vi "Cap_vs_RF-power.vi"() -> ()   [LabVIEW 2020]
uses:
  <vilib>/Utility/file.llb/Write Delimited Spreadsheet (string).vi
  <instrlib>/Agilent 428X Series/Agilent 428X Series.lvlib
  <instrlib>/Agilent PSG MXG Series/Agilent PSG MXG Series.lvlib
panel:
  in  "Register arrays":string[](array[string])
  in  "file path (dialog if empty)":path
  out "error out":errorcluster
  out "Array":string[][](array[string])
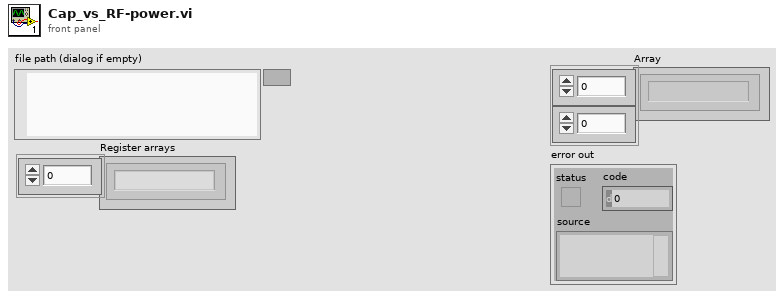
[diagram p1: front panel]
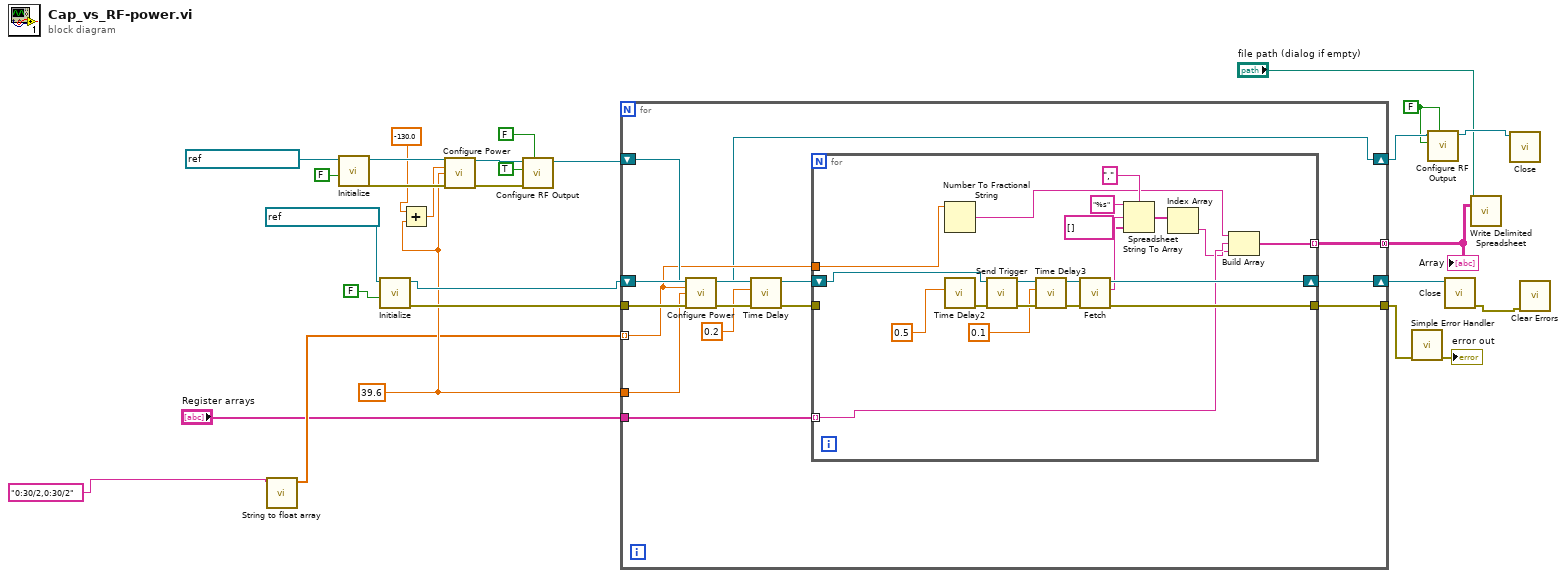
[diagram p0: block diagram]
diagram:
  w17 = FALSE ("Enable Modulation (T:Enable)")
  w6 = 39.6 ("Power Offset (0 dB)")
  n1 = call "String to float array.vi"("String"="0:30/2,0:30/2" ("Capa values")) -> ("Array - Numeric"=w2:dbl[])  [unwired: 9 in, 1 out]
  n2 = call <instrlib>:"Initialize.vi"("Reset (True)"=FALSE, "VISA resource name"=refnum<visa-resource-name> "GPIB0::30::INSTR") -> ("error out"=w10:errorcluster, "VISA resource name out"=w13:refnum<visa-resource-name>)  [unwired: 8 in]
  n3 = call <instrlib>:"Initialize.vi"("Reset (T: Reset)"=FALSE, "VISA resource name"=refnum<visa-resource-name> "GPIB0::17::INSTR") -> ("error out"=w8:errorcluster, "VISA resource name out"=w9:refnum<visa-resource-name>)  [unwired: 8 in]
  n4 = Add(x=-130.0 ("Power (-130 dBm)"), y=w6) -> (x+y=w5:dbl)
  n5 = call <instrlib>:"Configure Power.vi"("VISA resource name"=w13, "Power (-130 dBm)"=w5, "Power Offset (0 dB)"=w6, "error in (no error)"=w10) -> ("VISA resource name out"=w16:refnum<visa-resource-name>, "error out"=w11:errorcluster)  [unwired: 10 in]
  n6 = call <instrlib>:"Configure RF Output.vi"("Enable Modulation (T:Enable)"=FALSE, "error in (no error)"=w11, "Enable RF Output (F:Disable)"=TRUE, "VISA resource name"=w16) -> ("VISA resource name out"=w12:refnum<visa-resource-name>)  [unwired: 6 in, 1 out]
  n7 = for {
    shift-right: [w40] -> w26
    shift-left: w9 -> [w41]
    tunnel: "Register arrays" -> [w38]
    tunnel: w6 -> [w35]
    tunnel: w2 -> [w30] mode=indexing
    tunnel: [w31] -> w20 mode=concatenating
    shift-right: [w29] -> w19
    shift-left: w12 -> [w36]
    tunnel: w8 -> [w37]
    tunnel: [w39] -> w23
    n8 = call <instrlib>:"Configure Power.vi"("VISA resource name"=w36, "Power (-130 dBm)"=w30, "Power Offset (0 dB)"=w35, "error in (no error)"=w37) -> ("VISA resource name out"=w29:refnum<visa-resource-name>, "error out"=w34:errorcluster)  [unwired: 10 in]
    n9 = call "Time Delay"("error in (no error)"=w34, "Delay Time (s)"=0.2) -> ("error out"=w33:errorcluster)  [unwired: 9 in]
    n10 = for {
      shift-right: [w58] -> w40
      shift-left: w41 -> [w59]
      tunnel: w38 -> [w48] mode=indexing
      tunnel: [w49] -> w31 mode=indexing
      tunnel: w30 -> [w46]
      tunnel: w33 -> [_]
      tunnel: [w57] -> w39
      n11 = Number To Fractional String(number=w46) -> (F-format string=w45:string)  [unwired: 3 in]
      n12 = call "Time Delay2"("Delay Time (s)"=0.5) -> ("error out"=w56:errorcluster)  [unwired: 10 in]
      n13 = call <instrlib>:"Send Trigger.vi"("error in (no error)"=w56, "VISA resource name"=w59) -> ("error out"=w44:errorcluster, "VISA resource name out"=w60:refnum<visa-resource-name>)  [unwired: 8 in]
      n14 = call "Time Delay3"("error in (no error)"=w44, "Delay Time (s)"=0.1) -> ("error out"=w43:errorcluster)  [unwired: 9 in]
      n15 = call <instrlib>:"Fetch.vi"("error in (no error)"=w43, "VISA resource name"=w60) -> ("error out"=w57:errorcluster, "Returned Data"=w54:string, "VISA resource name out"=w58:refnum<visa-resource-name>)  [unwired: 7 in]
      n16 = Spreadsheet String To Array(delimiter (Tab)=",", format string="%s", spreadsheet string=w54, array type (2D Dbl)=string[] []) -> (array=w52:string[])
      n17 = Index Array(array=w52) -> (element=w47:string)  [unwired: 1 in]
      n18 = Build Array(w45, w48, w47) -> (w49:string[])
    }
  }
  "Array" <- w20
  n19 = call <vilib>:"Simple Error Handler.vi"("error in (no error)"=w23) -> ("error out"=→"error out":errorcluster)  [unwired: 4 in, 4 out]
  n20 = call <instrlib>:"Configure RF Output.vi"("Enable Modulation (T:Enable)"=w17, "Enable RF Output (F:Disable)"=w17, "VISA resource name"=w19) -> ("VISA resource name out"=w18:refnum<visa-resource-name>)  [unwired: 7 in, 1 out]
  n21 = call <instrlib>:"Close.vi"("VISA resource name"=w26) -> ("error out"=w21:errorcluster)  [unwired: 10 in]
  n22 = call-poly <vilib>:"Write Delimited Spreadsheet.vi"("file path (dialog if empty)"="file path (dialog if empty)", "2D data"=w20) -> ()  [unwired: 12 in, 2 out]
  n23 = call <instrlib>:"Close.vi"("VISA resource name"=w18) -> ()  [unwired: 10 in, 1 out]
  n24 = call <vilib>:"Clear Errors.vi"("error in (no error)"=w21) -> ()  [unwired: 5 in, 2 out]
